vi "5. CoffeeMaker Timing.vi"() -> ()   [LabVIEW 2018]
doc: "Coffee Machine Version 1.0: timing issues added"
uses:
  Controls/States.ctl
  <vilib>/Utility/file.llb/Read Delimited Spreadsheet (string).vi
panel:
  out "s? t:f":enum16{"next state", "current state"}(ring)
  out "error out":errorcluster
  in  "error in (no error)":errorcluster
  in  "Power Switch":bool
  in  "Simulation":cluster{"Water":dbl, "Coffee":dbl, "Milk":dbl} caption="Wasser" {"Milk" scale=0.0..100.0; "Water" scale=0.0..100.0; "Coffee" scale=0.0..100.0}
  out "Display":T1 {"Coffee" scale=0.0..80.0; "Brewing Chamber" scale=0.0..80.0}
  in  "Coffee Selection":T2 {"Type" min=0 max=2 scale=0.0..2.0}
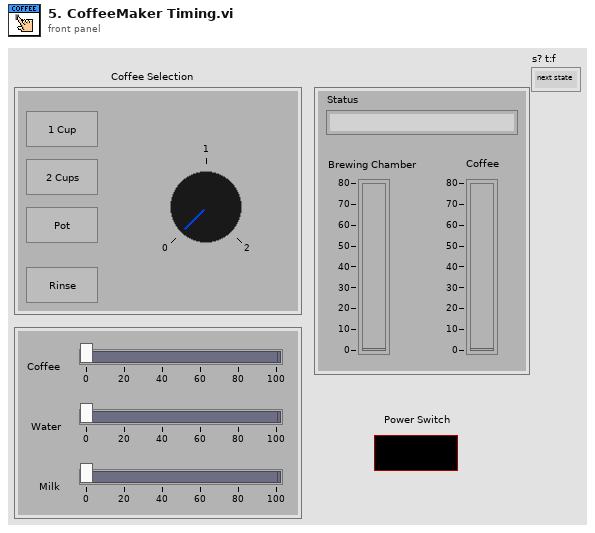
[diagram p1: front panel]
types:
  T1 = cluster{"Brewing Chamber":dbl, "Coffee":dbl, "Status":string}
  T2 = cluster{"1 Cup":bool, "2 Cups":bool, "Pot":bool, "Rinse":bool, "Type":i8}
  T3 = typedef "States.ctl" = enum16{"Initialize", "Set Language", "Wait for Power On", "Heat up", "Check and Wait for Water", "Rinsing", "Check Resources", "User Input", "Grinding", "Boiling", "Pouring", "Rinse before Stop", "Write Data", "Stop"}
  T4 = cluster{"Coffee":refnum<vi>, "Water":refnum<vi>, "Milk":refnum<vi>}
  T5 = cluster{"Status":refnum<vi>, "Brewing Chamber":refnum<vi>, "Coffee":refnum<vi>, "Power Switch":refnum<vi>}
  T6 = cluster{"Coffee Selection":refnum<vi>, "1 Cup":refnum<vi>, "2 Cups":refnum<vi>, "Pot":refnum<vi>, "Rinse":refnum<vi>, "Type":refnum<vi>}
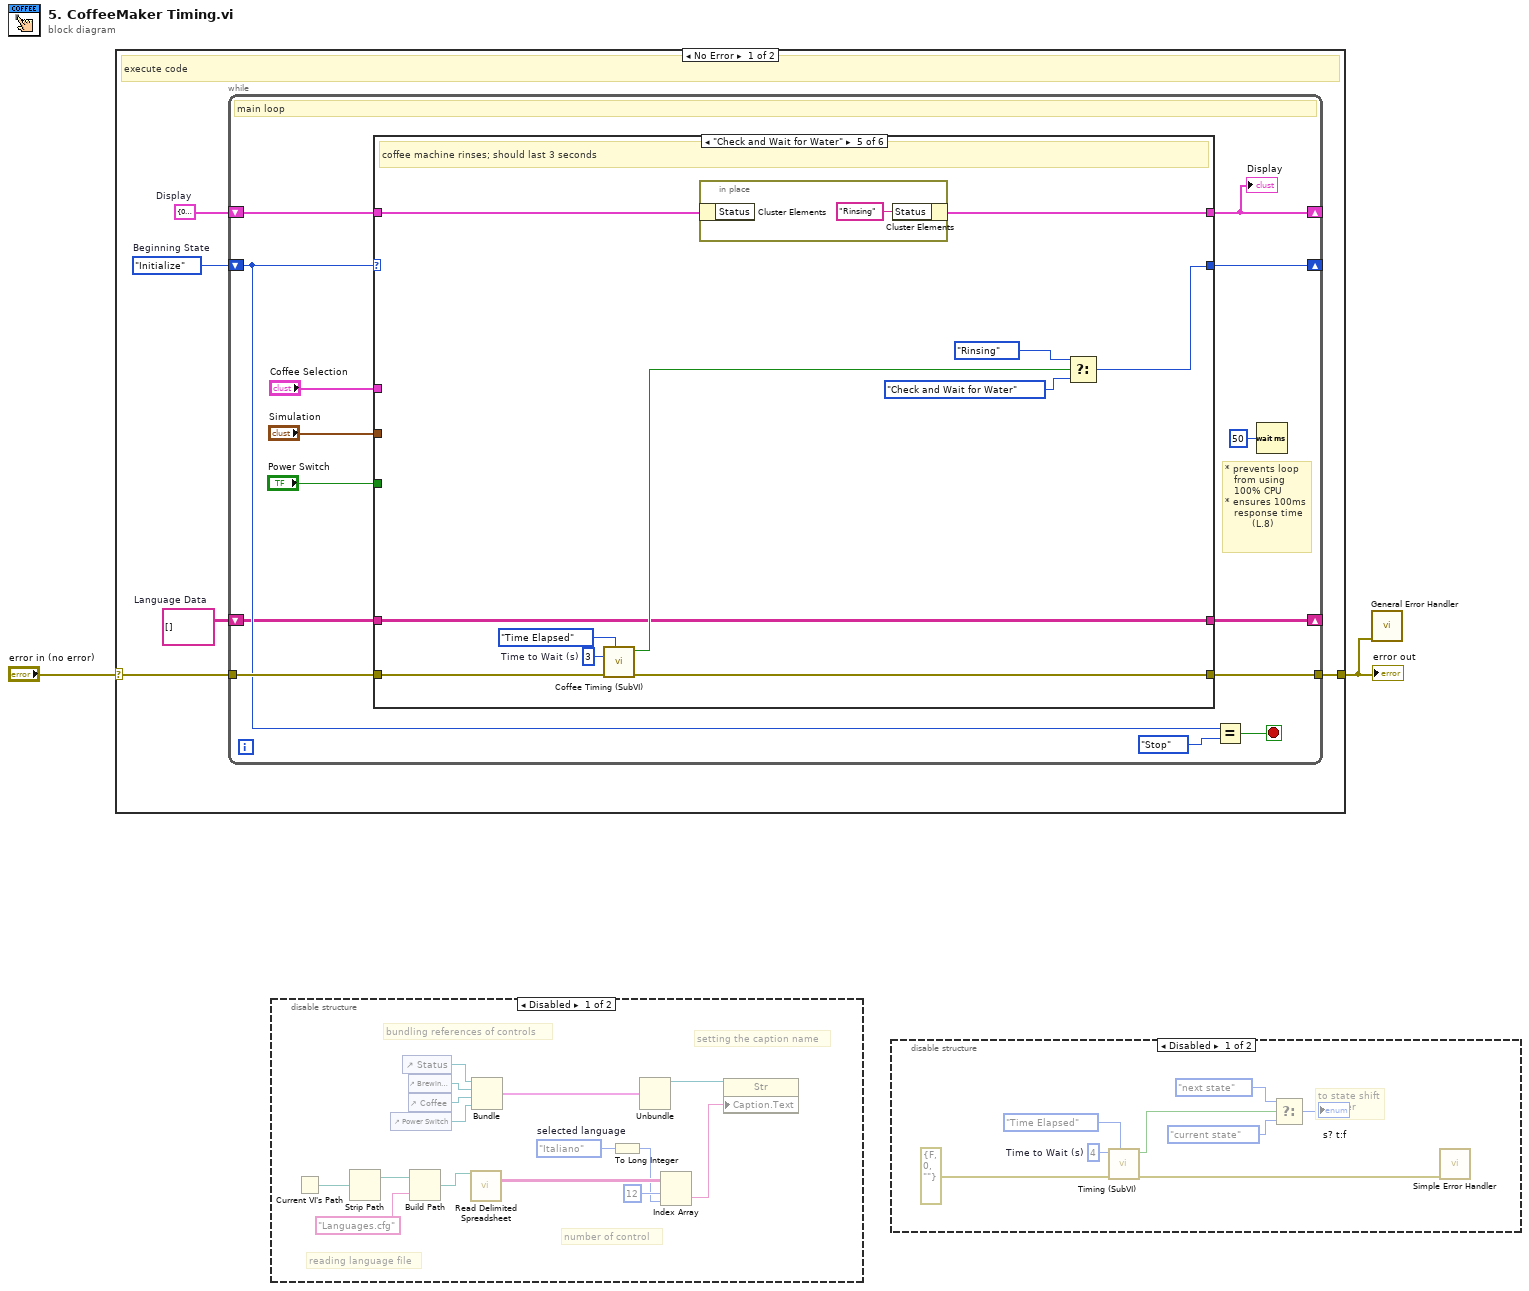
[diagram p0: block diagram]
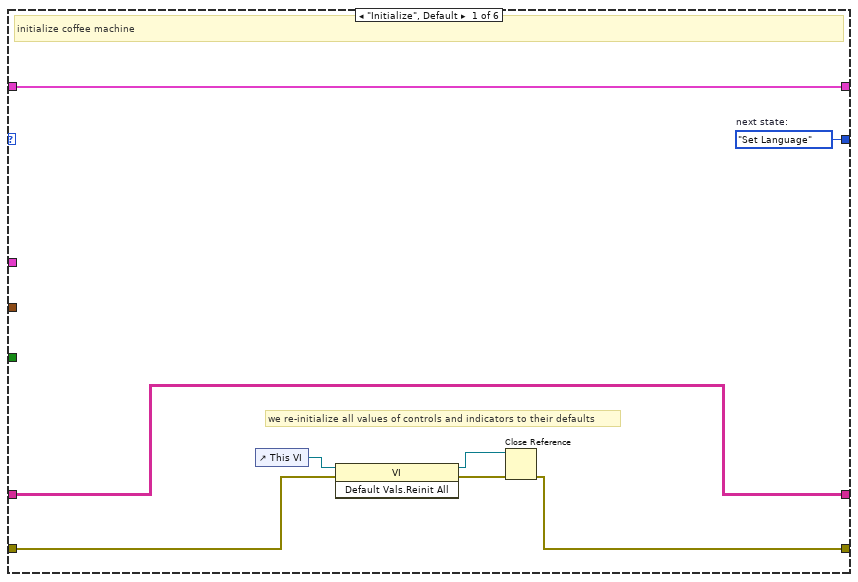
[diagram p4: hidden frame]
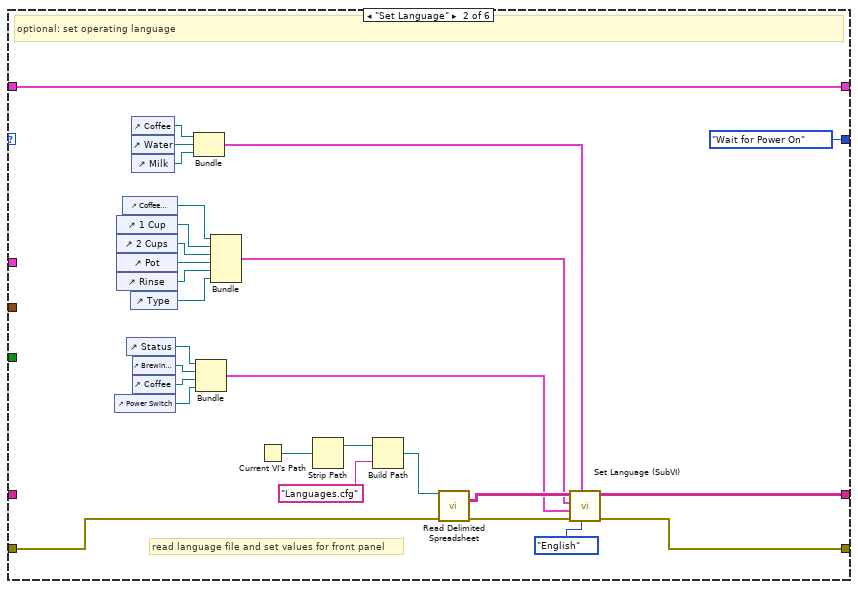
[diagram p5: hidden frame]
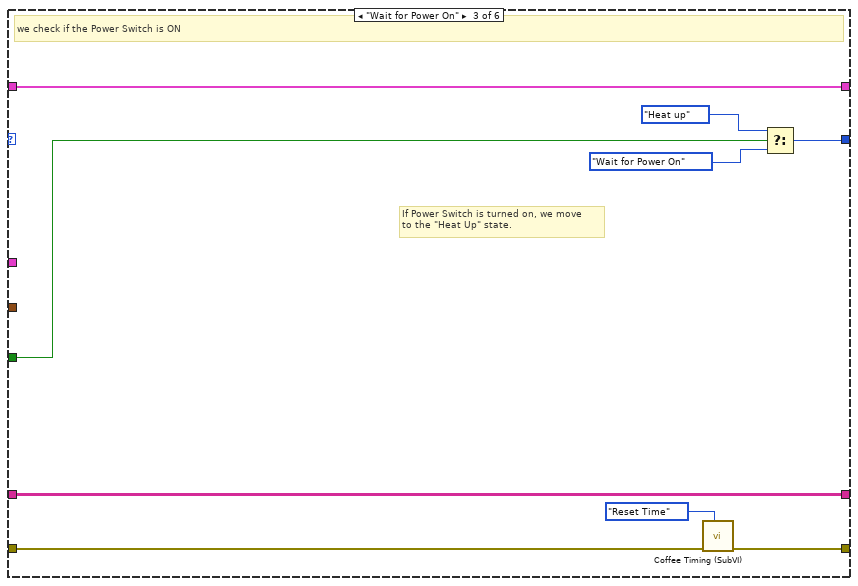
[diagram p6: hidden frame]
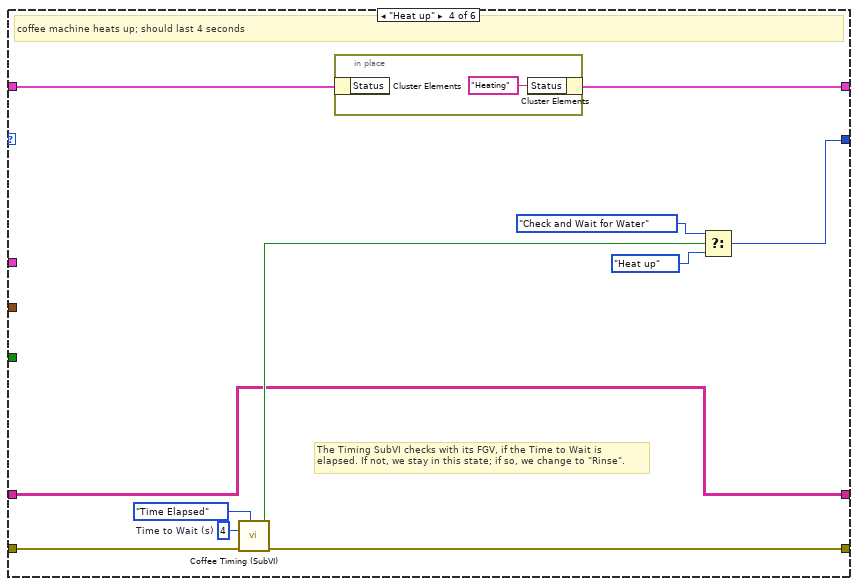
[diagram p7: hidden frame]
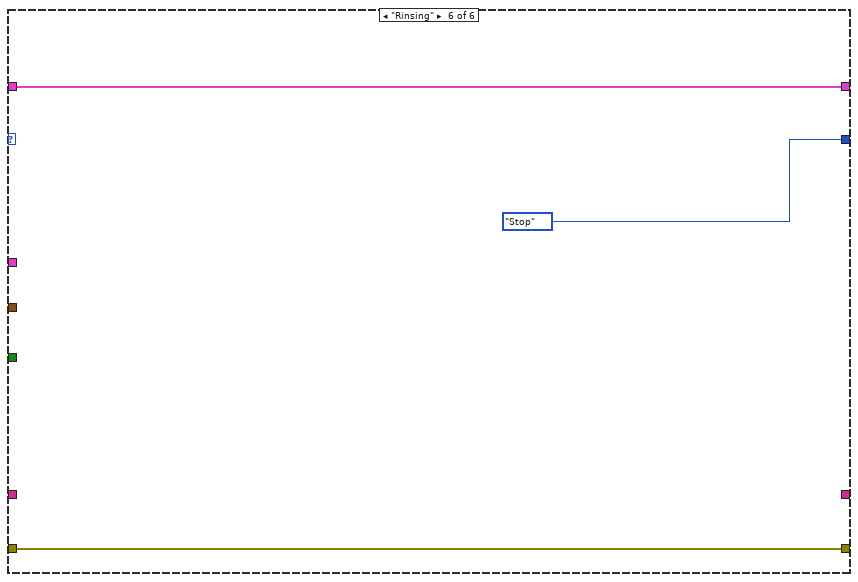
[diagram p8: hidden frame]
diagram:
  n1 = case shown="No Error" "error in (no error)" {
    selector: "error in (no error)" -> [w6 w94]
    tunnel: [w7 w94] -> w1
    frame No Error {
      w3 = string[][] []  # Language Data
      w4 = T1 {"Brewing Chamber"=0.0, "Coffee"=0.0, "Status"=""}  # Display
      w5 = States."Initialize"  # Beginning State
      # "execute code"
      n2 = while {
        tunnel: [w21] -> w7
        tunnel: w6 -> [w20]
        shift-right: [w18] -> _
        shift-left: w5 -> [w17]
        shift-right: [w11] -> _
        shift-left: w3 -> [w9]
        shift-right: [w10] -> _
        shift-left: w4 -> [w14]
        stop <- w15 stop-if-true
        # "* prevents loop\n   from using\n   100% CPU\n* ensures 100ms\n   response time\n         (L.8)"
        # "main loop"
        n3 = case shown="\"Check and Wait for Water\"" w17 {
          tunnel: [w23 w50 w59 w76 w88 w93] -> w21
          tunnel: w20 -> [w28 w51 w60 w77 w89 w93]
          tunnel: "Power Switch" -> [_ _ w66 _ _ _]
          tunnel: [w25 States."Wait for Power On" ("f") w65 w73 w85 States."Stop" ("f")] -> w18
          tunnel: [w24 w42 w62 w68 w79 w91] -> w10
          tunnel: w14 -> [w24 w42 w62 w69 w80 w91]
          tunnel: "Coffee Selection" -> [_ _ _ _ _ _]
          tunnel: "Simulation" -> [_ _ _ _ _ _]
          tunnel: [w22 w49 w61 w67 w81 _] -> w11
          tunnel: w9 -> [w22 _ w61 w67 w81 _]
          frame "Initialize", Default {
            w25 = States."Set Language"  # next state:
            # "we re-initialize all values of controls and indicators to their defaults"
            # "initialize coffee machine"
            n4 = control-ref of="This VI"() -> (w29:refnum<vi>)
            n5 = invoke class="VI" method="Default Vals.Reinit All"(reference=w29, error in=w28) -> (reference out=w27:refnum<vi>, error out=w26:errorcluster)  [unwired: 1 in, 1 out]
            n6 = Close Reference(reference=w27, error in (no error)=w26) -> (error out=w23:errorcluster)
          }
          frame "Set Language" {
            # "read language file and set values for front panel"
            # "optional: set operating language"
            n7 = control-ref of="Power Switch"() -> (w32:refnum<vi>)
            n8 = control-ref of="1 Cup"() -> (w40:refnum<vi>)
            n9 = control-ref of="2 Cups"() -> (w39:refnum<vi>)
            n10 = control-ref of="Pot"() -> (w38:refnum<vi>)
            n11 = control-ref of="Rinse"() -> (w37:refnum<vi>)
            n12 = control-ref of="Coffee Selection"() -> (w41:refnum<vi>)
            n13 = control-ref of="Status"() -> (w35:refnum<vi>)
            n14 = control-ref of="Type"() -> (w36:refnum<vi>)
            n15 = control-ref of="Coffee"() -> (w46:refnum<vi>)
            n16 = control-ref of="Water"() -> (w45:refnum<vi>)
            n17 = control-ref of="Milk"() -> (w44:refnum<vi>)
            n18 = control-ref of="Brewing Chamber"() -> (w34:refnum<vi>)
            n19 = control-ref of="Coffee"() -> (w33:refnum<vi>)
            n20 = Bundle("Coffee"=w46, "Water"=w45, "Milk"=w44) -> (w48:T4)  [unwired: 1 in]
            n21 = Bundle("Status"=w35, "Brewing Chamber"=w34, "Coffee"=w33, "Power Switch"=w32) -> (w30:T5)  [unwired: 1 in]
            n22 = Bundle("Coffee Selection"=w41, "1 Cup"=w40, "2 Cups"=w39, "Pot"=w38, "Rinse"=w37, "Type"=w36) -> (w31:T6)  [unwired: 1 in]
            n23 = Current VI's Path() -> (path=w52:path)
            n24 = Strip Path(path=w52) -> (stripped path=w53:path)  [unwired: 1 out]
            n25 = Build Path(base path=w53, name or relative path="Languages.cfg") -> (appended path=w55:path)
            n26 = call-poly <vilib>:"Read Delimited Spreadsheet.vi"("file path (dialog if empty)"=w55, "error in (no error)"=w51) -> ("all rows"=w57:string[][], "error out"=w56:errorcluster)  [unwired: 8 in, 4 out]
            n27 = call "Set Language (SubVI).vi"("Language (English)"=enum16{"English", "Deutsch", "Italiano"}."English" ("Language"), "Simulation \nReferences"=w48, "error in (no error)"=w56, "Status\nReferences"=w30, "Selection \nReferences"=w31, "Language Data"=w57) -> ("error out"=w50:errorcluster, "Language Data Out"=w49:string[][])  [unwired: 4 in]
          }
          frame "Wait for Power On" {
            # "If Power Switch is turned on, we move\nto the \"Heat Up\" state."
            # "we check if the Power Switch is ON"
            n28 = call "Coffee Timing (SubVI).vi"("Function"=enum16{"Reset Time", "Time Elapsed"}."Reset Time", "error in (no error)"=w60) -> ("error out"=w59:errorcluster)  [unwired: 7 in, 2 out]
            n29 = Select(t=States."Heat up" ("Beginning State"), s=w66, f=States."Wait for Power On") -> (s? t:f=w65:T3)
          }
          frame "Heat up" {
            w74 = 4  # Time to Wait (s)
            # "The Timing SubVI checks with its FGV, if the Time to Wait is\nelapsed. If not, we stay in this state; if so, we change to \"Rinse\"."
            # "coffee machine heats up; should last 4 seconds"
            n30 = call "Coffee Timing (SubVI).vi"("Function"=enum16{"Reset Time", "Time Elapsed"}."Time Elapsed", "error in (no error)"=w77, "Time to Wait (s)"=w74) -> ("error out"=w76:errorcluster, "Time elapsed ?"=w70:bool)  [unwired: 6 in, 1 out]
            n31 = in-place {
              n32 = in-place-cluster #1(w69) -> ()  [unwired: 1 out]
              n33 = in-place-cluster #1("Status"="Heating") -> (w68:T1)
            }
            n34 = Select(t=States."Check and Wait for Water" ("Beginning State"), s=w70, f=States."Heat up" ("Beginning State")) -> (s? t:f=w73:T3)
          }
          frame "Check and Wait for Water" {
            w86 = 3  # Time to Wait (s)
            # "coffee machine rinses; should last 3 seconds"
            n35 = call "Coffee Timing (SubVI).vi"("Function"=enum16{"Reset Time", "Time Elapsed"}."Time Elapsed", "error in (no error)"=w89, "Time to Wait (s)"=w86) -> ("error out"=w88:errorcluster, "Time elapsed ?"=w82:bool)  [unwired: 6 in, 1 out]
            n36 = in-place {
              n37 = in-place-cluster #2(w80) -> ()  [unwired: 1 out]
              n38 = in-place-cluster #2("Status"="Rinsing") -> (w79:T1)
            }
            n39 = Select(t=States."Rinsing" ("Beginning State"), s=w82, f=States."Check and Wait for Water" ("Beginning State")) -> (s? t:f=w85:T3)
          }
          frame "Rinsing" {
          }
        }
        "Display" <- w10
        n40 = Equal?(x=w17, y=States."Stop") -> (x = y?=w15:bool)
        n41 = Wait (ms)(milliseconds to wait=u32 50) -> ()  [unwired: 1 out]
      }
    }
    frame Error {
      # "do nothing"
    }
  }
  "error out" <- w1
  n42 = disable-structure shown="Disabled" {
    frame Disabled {
      w97 = enum16{"English", "Deutsch", "Italiano"}."Italiano"  # selected language
      # "setting the caption name"
      # "number of control"
      # "reading language file"
      # "bundling references of controls"
      n43 = Current VI's Path() -> (path=w103:path)
      n44 = Strip Path(path=w103) -> (stripped path=w102:path)  [unwired: 1 out]
      n45 = control-ref of="Power Switch"() -> (w109:refnum<vi>)
      n46 = control-ref of="Status"() -> (w106:refnum<vi>)
      n47 = control-ref of="Brewing Chamber"() -> (w107:refnum<vi>)
      n48 = control-ref of="Coffee"() -> (w108:refnum<vi>)
      n49 = Build Path(base path=w102, name or relative path="Languages.cfg") -> (appended path=w100:path)
      n50 = call-poly <vilib>:"Read Delimited Spreadsheet.vi"("file path (dialog if empty)"=w100) -> ("all rows"=w99:string[][])  [unwired: 9 in, 5 out]
      n51 = Bundle("Status"=w106, "Brewing Chamber"=w107, "Coffee"=w108, "Power Switch"=w109) -> (w105:T5)  [unwired: 1 in]
      n52 = To Long Integer(number=w97) -> (32bit integer=w96:i32)
      n53 = Unbundle(w105) -> ("Status"=w104:refnum<vi>)  [unwired: 3 out]
      n54 = Index Array(array=w99, index (row)=12, index (col)=w96) -> (element=w95:string)
      n55 = property class="Str"(reference=w104, "Caption.Text"=w95) -> ()  [unwired: 1 in, 2 out]
    }
    frame Enabled {
    }
  }
  n56 = disable-structure shown="Disabled" {
    frame Disabled {
      w116 = 4  # Time to Wait (s)
      # "to state shift\nregister"
      n57 = call "Timing (SubVI).vi"("Function"=enum16{"Reset Time", "Time Elapsed"}."Time Elapsed", "error in (no error)"=errorcluster {"status"=FALSE, "code"=0, "source"=""}, "Time to Wait (s)"=w116) -> ("error out"=w114:errorcluster, "Time elapsed ?"=w113:bool)  [unwired: 6 in, 1 out]
      n58 = Select(t=enum16{"next state", "current state"}."next state", s=w113, f=enum16{"next state", "current state"}."current state") -> (s? t:f=→"s? t:f":enum16{"next state", "current state"})
      n59 = call <vilib>:"Simple Error Handler.vi"("error in (no error)"=w114) -> ()  [unwired: 4 in, 5 out]
    }
    frame Enabled {
    }
  }
  n60 = call <vilib>:"General Error Handler.vi"("error in (no error)"=w1) -> ()  [unwired: 10 in, 5 out]
